vi "Set Tester Rx.vi"(8 "error in (no error)":errorcluster, 10 "Tester Rx":refnum<vi>, 11 "PLC Sim Controller Actor in":refnum<class "PLC Sim Controller Actor.lvclass">) -> (0 "error out":errorcluster, 3 "PLC Sim Controller Actor out":refnum<class "PLC Sim Controller Actor.lvclass">)   [LabVIEW 2019]
uses:
  PLC Sim Controller Actor.lvclass
  C:/Program Files (x86)/National Instruments/LabVIEW 2019/vi.lib/ActorFramework/Actor/Actor.lvclass
  <vilib>/ActorFramework/Message Enqueuer/Message Enqueuer.lvclass
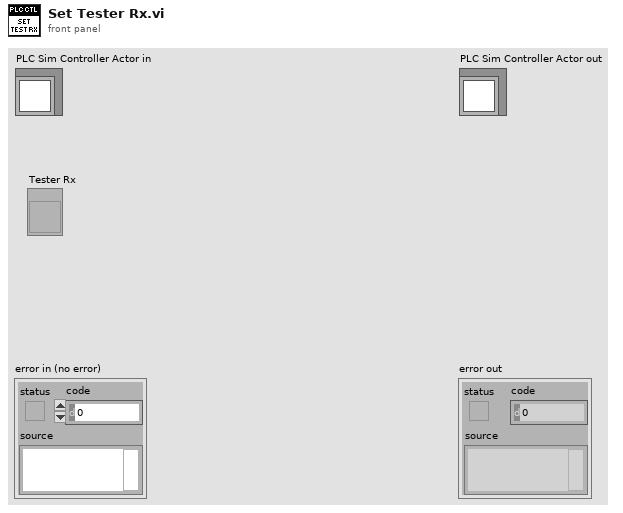
[diagram p1: front panel]
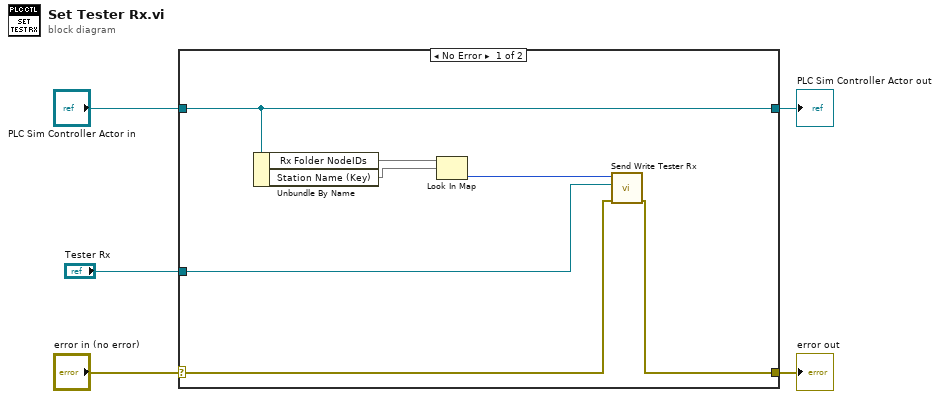
[diagram p0: block diagram]
diagram:
  n1 = case shown="No Error" "error in (no error)" {
    selector: "error in (no error)" -> [w10 w14]
    tunnel: [w9 w14] -> w4
    tunnel: [w12 w13] -> w2
    tunnel: "PLC Sim Controller Actor in" -> [w12 w13]
    tunnel: "Tester Rx" -> [w11 _]
    frame No Error {
      n2 = Unbundle By Name(w12) -> ("Rx Folder NodeIDs"=w8, "Station Name (Key)"=w7)
      n3 = Look In Map(map=w8, key=w7) -> (value=w6:i32)  [unwired: 1 in, 1 out]
      n4 = call "Send Write Tester Rx.vi"("error in (no error)"=w10, "Tester Rx"=w11, "Message Enqueuer"=w6) -> ("error out"=w9:errorcluster)  [unwired: 7 in, 1 out]
    }
    frame Error {
    }
  }
  "error out" <- w4
  "PLC Sim Controller Actor out" <- w2
